vi "Fill.vi"(6 "Color":u32(colorbox), 8 "error in (no error)":errorcluster, 9 "point(x,y)":cluster{"x":i16, "y":i16}, 10 "Ref Color":u32(colorbox), 11 "Data in":T1={"Class"={"Ants"=refnum, "Layer"=refnum, "Templates"=refnum, "Icon"=refnum, "Glyph"=refnum, "Settings"=refnum, "Tools"=refnum, "History"=refnum}, "Ref"={"Add Layer"=refnum, "Remove Layer"=refnum, "Line Text"=[], "Body Text Spec"=refnum, "DNL_Font"=refnum, "glyph path str"=refnum, "templates path str"=refnum, "Arrow Up"=refnum, "Arrow Down"=refnum, "IE VI Ref"=refnum, "Glyphs tree"=refnum, "Templates tree"=refnum, "Layer Icon Text"=refnum, "Layer Template"=refnum, "Body Text"=refnum, "Search Templates"=refnum, "TextMarker"=refnum, "Tab Control"=refnum, "Search Glyphs"=refnum, "Line Color"=refnum, "DNL_Glyphs []"=refnum, "Fill Color"=refnum, "Tools"=refnum, "Icon"=refnum, "Preview"=refnum, "Ants"=refnum, "Terminals"=refnum, "menu reference"=refnum, "LayerNames"=[], "GlyphLoadAnimation"=refnum, "TemplateLoadAnimation"=refnum, "refreshGlyphs"=refnum, "refreshTemplates"=refnum}, "Support"={"AntsRect"={"left"=0, "top"=0, "right"=0, "bottom"=0}, "Mouse Move Coords"={"Horizontal"=0, "Vertical"=0}, "Mouse Down Coords"={"Horizontal"=0, "Vertical"=0}, "Temp Coord"={"Horizontal"=0, "Vertical"=0}, "Action"=enum."Default", "Edge Color"=4914962, "Fill Color"=16860, "Mouse Down?"=FALSE, "Draft Mode?"=FALSE, "Temp Icon"=bytes[3102], "CTRL Pressed"=FALSE, "Move Selection?"=FALSE, "AntsRect Orig"={"left"=0, "top"=0, "right"=0, "bottom"=0}, "Text"="", "TM Set?"=FALSE, "Mouse inside icon?"=FALSE, "Tool (old value)"=0, "Pencil Move Color"=0, "Swap Colors?"=FALSE, "Shift pressed?"=FALSE}}) -> (0 "error out":errorcluster, 3 "Data out":T1={"Class"={"Ants"=refnum, "Layer"=refnum, "Templates"=refnum, "Icon"=refnum, "Glyph"=refnum, "Settings"=refnum, "Tools"=refnum, "History"=refnum}, "Ref"={"Add Layer"=refnum, "Remove Layer"=refnum, "Line Text"=[], "Body Text Spec"=refnum, "DNL_Font"=refnum, "glyph path str"=refnum, "templates path str"=refnum, "Arrow Up"=refnum, "Arrow Down"=refnum, "IE VI Ref"=refnum, "Glyphs tree"=refnum, "Templates tree"=refnum, "Layer Icon Text"=refnum, "Layer Template"=refnum, "Body Text"=refnum, "Search Templates"=refnum, "TextMarker"=refnum, "Tab Control"=refnum, "Search Glyphs"=refnum, "Line Color"=refnum, "DNL_Glyphs []"=refnum, "Fill Color"=refnum, "Tools"=refnum, "Icon"=refnum, "Preview"=refnum, "Ants"=refnum, "Terminals"=refnum, "menu reference"=refnum, "LayerNames"=[], "GlyphLoadAnimation"=refnum, "TemplateLoadAnimation"=refnum, "refreshGlyphs"=refnum, "refreshTemplates"=refnum}, "Support"={"AntsRect"={"left"=0, "top"=0, "right"=0, "bottom"=0}, "Mouse Move Coords"={"Horizontal"=0, "Vertical"=0}, "Mouse Down Coords"={"Horizontal"=0, "Vertical"=0}, "Temp Coord"={"Horizontal"=0, "Vertical"=0}, "Action"=enum."Default", "Edge Color"=4914962, "Fill Color"=16860, "Mouse Down?"=FALSE, "Draft Mode?"=FALSE, "Temp Icon"=bytes[3102], "CTRL Pressed"=FALSE, "Move Selection?"=FALSE, "AntsRect Orig"={"left"=0, "top"=0, "right"=0, "bottom"=0}, "Text"="", "TM Set?"=FALSE, "Mouse inside icon?"=FALSE, "Tool (old value)"=0, "Pencil Move Color"=0, "Swap Colors?"=FALSE, "Shift pressed?"=FALSE}})   [LabVIEW 2020, in "Tools Paint.lvclass"]
uses:
  Tools Paint.lvclass
  Ants/Ants.lvclass
  FakedArray/FakedArray.lvclass
  vi.lib/LabVIEW Icon API/lv_icon/Classes/Icon/Icon.lvclass
  Icon Library/Glyph.lvclass
  Settings/Settings.lvclass
  History/History/History.lvclass
  vi.lib/LabVIEW Icon API/lv_icon/Classes/Layer/Layer.lvclass
  vi.lib/LabVIEW Icon API/lv_icon/Classes/Icon Framework/Icon Framework.lvclass
  Tools Paint.lvclass/Tools Paint.ctl
  lv_icon.lvlib
  vi.lib/LabVIEW Icon API/lv_icon/Controls/LayerType.ctl
  vi.lib/LabVIEW Icon API/LabVIEW Icon API.lvlib
  <vilib>/Utility/miscctls.llb/LVPoint32TypeDef.ctl
  Controls/SupportClass_Action.ctl
  vi.lib/LabVIEW Icon API/lv_icon/Controls/IEColor.ctl
  Controls/Support Cluster.ctl
  Controls/References Cluster.ctl
  Controls/IE Classes.ctl
  Controls/Global Data.ctl
panel:
  in  "Fill":string="Fill"
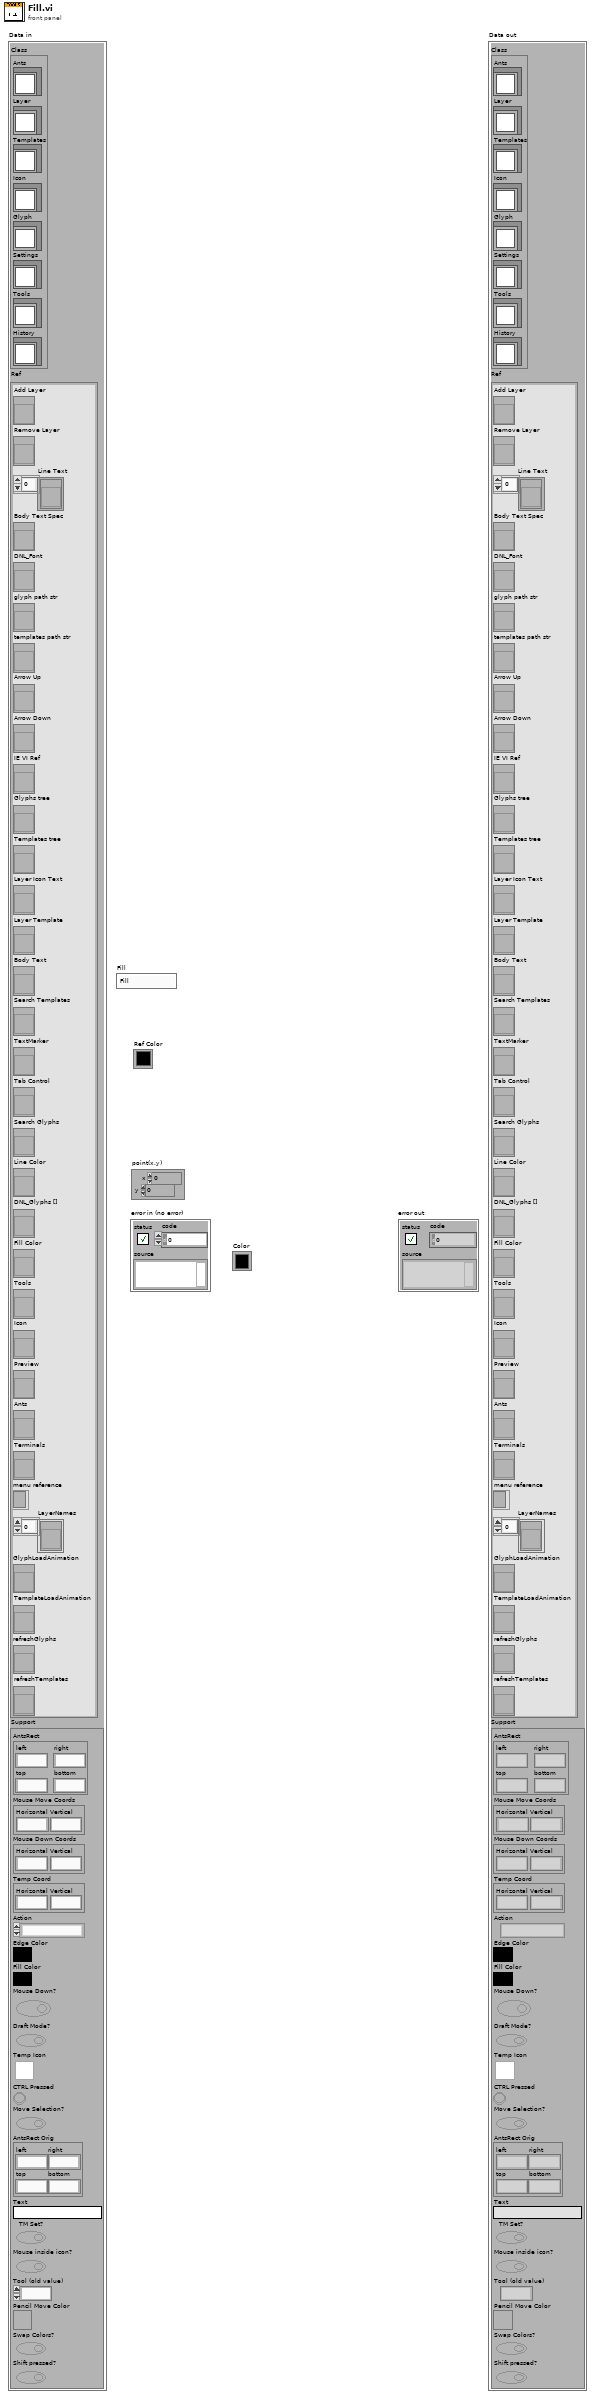
[diagram p1: front panel]
types:
  T1 = typedef "lv_icon.lvlib/Global Data.ctl" = cluster{"Class":T2, "Ref":T3, "Support":T4}
  T2 = typedef "lv_icon.lvlib/IE Classes.ctl" = cluster{"Ants":refnum<class "Ants.lvclass">, "Layer":refnum<class "FakedArray.lvclass">, "Templates":refnum<class "FakedArray.lvclass">, "Icon":refnum<class "Icon.lvclass">, "Glyph":refnum<class "Glyph.lvclass">, "Settings":refnum<class "Settings.lvclass">, "Tools":refnum<class "Tools Paint.lvclass">, "History":refnum<class "History.lvclass">}
  T3 = typedef "lv_icon.lvlib/References Cluster.ctl" = cluster{"Add Layer":refnum<vi>, "Remove Layer":refnum<vi>, "Line Text":refnum<vi>[], "Body Text Spec":refnum<vi>, "DNL_Font":refnum<vi>, "glyph path str":refnum<vi>, "templates path str":refnum<vi>, "Arrow Up":refnum<vi>, "Arrow Down":refnum<vi>, "IE VI Ref":refnum<vi>, "Glyphs tree":refnum<vi>, "Templates tree":refnum<vi>, "Layer Icon Text":refnum<vi>, "Layer Template":refnum<vi>, "Body Text":refnum<vi>, "Search Templates":refnum<vi>, "TextMarker":refnum<vi>, "Tab Control":refnum<vi>, "Search Glyphs":refnum<vi>, "Line Color":refnum<vi>, "DNL_Glyphs []":refnum<vi>, "Fill Color":refnum<vi>, "Tools":refnum<vi>, "Icon":refnum<vi>, "Preview":refnum<vi>, "Ants":refnum<vi>, "Terminals":refnum<vi>, "menu reference":refnum<k9>, "LayerNames":refnum<vi>[], "GlyphLoadAnimation":refnum<vi>, "TemplateLoadAnimation":refnum<vi>, "refreshGlyphs":refnum<vi>, "refreshTemplates":refnum<vi>}
  T4 = typedef "lv_icon.lvlib/Support Cluster.ctl" = cluster{"AntsRect":cluster{"left":i16, "top":i16, "right":i16, "bottom":i16}, "Mouse Move Coords":T5, "Mouse Down Coords":T5, "Temp Coord":T5, "Action":T6, "Edge Color":T7, "Fill Color":T7, "Mouse Down?":bool, "Draft Mode?":bool, "Temp Icon":picture, "CTRL Pressed":bool, "Move Selection?":bool, "AntsRect Orig":cluster{"left":i16, "top":i16, "right":i16, "bottom":i16}, "Text":string, "TM Set?":bool, "Mouse inside icon?":bool, "Tool (old value)":u32, "Pencil Move Color":u32, "Swap Colors?":bool, "Shift pressed?":bool}
  T5 = typedef "LVPoint32TypeDef.ctl" = cluster{"Horizontal":i32, "Vertical":i32}
  T6 = typedef "SupportClass_Action.ctl" = enum16{"Default", "Move Selection", "Glyph Library", "Tool"}
  T7 = typedef "IEColor.ctl" = u32
  T8 = typedef "LayerType.ctl" = enum16{"Graphic", "Text", "Tool", "Graphic Drop"}
  T9 = typedef "lv_icon.lvlib/INI Data.ctl" = cluster{"Show Terminals?":bool, "Text":cluster{"Font":T10, "Alignment":T11, "Size":T12}, "3rd party Templates":cluster{"Store 3rd party Templates?":bool, "Folder Name":string}, "Merge user layers on commit":bool, "Body Text":T13, "Fill Color":T7, "Edge Color":T7, "Tab":u16, "Tool":T14, "Disable Layers?":bool}
  T10 = typedef "Font.ctl" = string
  T11 = typedef "Alignment.ctl" = u16
  T12 = typedef "Font Size.ctl" = u8
  T13 = typedef "BodyText.ctl" = cluster{"Line 1 text":string, "Line 2 text":string, "Line 3 text":string, "Line 4 text":string, "Line 1 color":u32, "Line 2 color":u32, "Line 3 color":u32, "Line 4 color":u32, "Body Text Spec":cluster{"Font":T10, "Alignment":T11, "Size":u8}, "Center text vertically":bool, "Capitalize Text":bool}
  T14 = typedef "Tools.ctl" = enum32{"Pencil", "Line", "Dropper", "Fill", "Rectangle", "Filled Rectangle", "Ellipse", "Filled Ellipse", "Eraser", "Text", "Select", "Move"}
  T15 = typedef "Layer.ctl" = cluster{"LayerIcon":picture, "LayerName":string, "Opacity":u8, "Visibility?":bool}
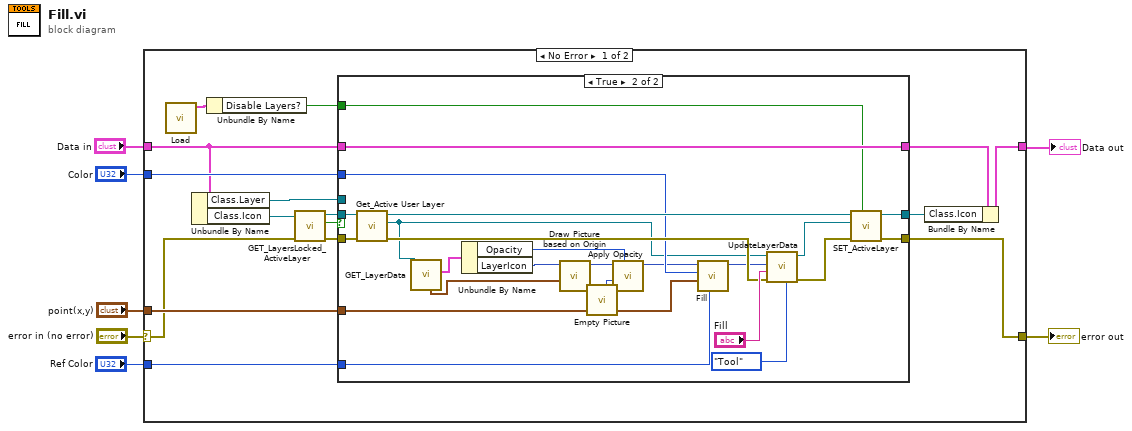
[diagram p0: block diagram]
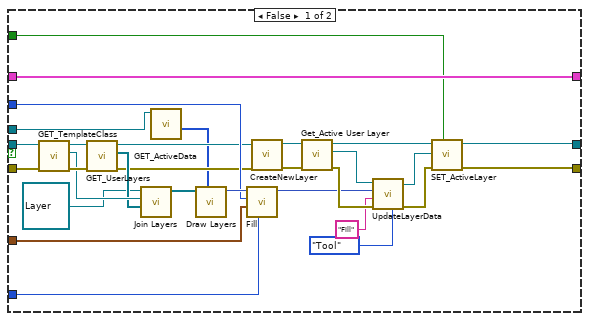
[diagram p2: hidden frame]
diagram:
  n1 = case shown="No Error" "error in (no error)" {
    selector: "error in (no error)" -> [w17 w79]
    tunnel: [w13 w79] -> w6
    tunnel: "point(x,y)" -> [w23 _]
    tunnel: "Color" -> [w19 _]
    tunnel: "Ref Color" -> [w18 _]
    tunnel: "Data in" -> [w15 w78]
    tunnel: [w12 w78] -> w1
    frame No Error {
      n2 = call "Load.vi"() -> ("INI Data"=w9:T9)  [unwired: 3 in, 8 out]
      n3 = Unbundle By Name(w15) -> ("Class.Layer"=w10:refnum<class "FakedArray.lvclass">, "Class.Icon"=w16:refnum<class "Icon.lvclass">)
      n4 = Unbundle By Name(w9) -> ("Disable Layers?"=w8:bool)
      n5 = call-dynamic "GET_LayersLocked_ActiveLayer.vi"("error in (no error)"=w17, "Icon.lvclass in"=w16) -> ("error out"=w21:errorcluster, "Layers Locked?"=w20:bool, "Icon.lvclass out"=w22:refnum<class "Icon.lvclass">)  [unwired: 7 out]
      n6 = case shown="True" w20 {
        tunnel: w23 -> [w44 w68]
        tunnel: [w30 w75] -> w11
        tunnel: w22 -> [w52 w77]
        tunnel: w21 -> [w53 w76]
        tunnel: w19 -> [w45 w69]
        tunnel: w18 -> [w46 w67]
        tunnel: [w28 w55] -> w13
        tunnel: w15 -> [w27 w56]
        tunnel: [w27 w56] -> w14
        tunnel: w10 -> [w25 _]
        tunnel: w8 -> [w26 w54]
        frame False {
          n7 = call-dynamic "GET_TemplateClass.vi"("error in (no error)"=w53, "Icon.lvclass in"=w52) -> ("error out"=w51:errorcluster, "Icon Framework.lvclass"=w49:refnum<class "Icon Framework.lvclass">, "Icon.lvclass out"=w50:refnum<class "Icon.lvclass">)  [unwired: 7 out]
          n8 = call-dynamic "GET_UserLayers.vi"("error in (no error)"=w51, "Icon.lvclass in"=w50) -> ("error out"=w32:errorcluster, "All Layers"=w43:refnum<class "Layer.lvclass">[], "Icon.lvclass out"=w33:refnum<class "Icon.lvclass">)  [unwired: 7 out]
          n9 = call "Join Layers.vi"("User Layers"=w43, "Template"=w49, "Icon Text"=refnum<class "Layer.lvclass"> refnum) -> ("Layer out"=w48:refnum<class "Layer.lvclass">[])  [unwired: 3 in, 5 out]
          n10 = call-dynamic "GET_ActiveData.vi"("FakedArray in"=w25) -> ("Active Data []"=w24:i32[])  [unwired: 5 in, 5 out]
          n11 = call "Draw Layers.vi"("Active User Layer Data []"=w24, "Layers"=w48) -> ("Picture"=w47:picture)  [unwired: 3 in, 6 out]
          n12 = call "Fill.vi"("Ref Color"=w46, "Pic Mouse Down"=w44, "New Color"=w45, "Pic In"=w47) -> ("Pic Out"=w31:picture)  [unwired: 3 in, 4 out]
          n13 = call "CreateNewLayer.vi"("error in"=w32, "Icon.lvclass"=w33) -> ("error out"=w41:errorcluster, "Icon.lvclass out"=w42:refnum<class "Icon.lvclass">)  [unwired: 3 in, 5 out]
          n14 = call-dynamic "Get_Active User Layer.vi"("error in (no error)"=w41, "Icon in"=w42) -> ("error out"=w36:errorcluster, "Layer.lvclass"=w40:refnum<class "Layer.lvclass">, "Icon out"=w39:refnum<class "Icon.lvclass">)  [unwired: 7 out]
          n15 = call "UpdateLayerData.vi"("Type"=LayerType."Tool", "error in"=w36, "LayerName"="Fill" ("FileName"), "new picture"=w31, "Active Layer"=w40) -> ("error out"=w37:errorcluster, "Layer.lvclass out"=w38:refnum<class "Layer.lvclass">)  [unwired: 3 in, 2 out]
          n16 = call-dynamic "SET_ActiveLayer.vi"("Combine User Layers?"=w26, "error in (no error)"=w37, "Layer.lvclass"=w38, "Icon.lvclass in"=w39) -> ("error out"=w28:errorcluster, "Icon.lvclass out"=w30:refnum<class "Icon.lvclass">)  [unwired: 6 out]
        }
        frame True {
          n17 = call-dynamic "Get_Active User Layer.vi"("error in (no error)"=w76, "Icon in"=w77) -> ("error out"=w71:errorcluster, "Layer.lvclass"=w62:refnum<class "Layer.lvclass">, "Icon out"=w74:refnum<class "Icon.lvclass">)  [unwired: 7 out]
          n18 = call-dynamic "GET_LayerData.vi"("Layer.lvclass in"=w62) -> ("Data"=w61:T15, "Origin"=w59:T5)  [unwired: 1 in, 8 out]
          n19 = Unbundle By Name(w61) -> ("Opacity"=w58:u8, "LayerIcon"=w60:picture)
          n20 = call "Draw Picture based on Origin.vi"("Origin"=w59, "LayerIcon in"=w60) -> ("LayerIcon out"=w63:picture)  [unwired: 1 in, 8 out]
          n21 = call "Empty Picture"() -> ("empty picture"=w64:picture)
          n22 = call "Apply Opacity.vi"("% (100)"=w58, "Bottom"=w64, "Top"=w63) -> ("new picture"=w57:picture)  [unwired: 8 out]
          n23 = call "Fill.vi"("Ref Color"=w67, "Pic Mouse Down"=w68, "New Color"=w69, "Pic In"=w57) -> ("Pic Out"=w66:picture)  [unwired: 3 in, 4 out]
          n24 = call "UpdateLayerData.vi"("Type"=LayerType."Tool", "error in"=w71, "LayerName"="Fill", "new picture"=w66, "Active Layer"=w62) -> ("error out"=w70:errorcluster, "Layer.lvclass out"=w65:refnum<class "Layer.lvclass">)  [unwired: 3 in, 2 out]
          n25 = call-dynamic "SET_ActiveLayer.vi"("Combine User Layers?"=w54, "error in (no error)"=w70, "Layer.lvclass"=w65, "Icon.lvclass in"=w74) -> ("error out"=w55:errorcluster, "Icon.lvclass out"=w75:refnum<class "Icon.lvclass">)  [unwired: 6 out]
        }
      }
      n26 = Bundle By Name(cluster=w14, "Class.Icon"=w11) -> (w12:T1)
    }
    frame Error {
    }
  }
  "error out" <- w6
  "Data out" <- w1
